vi "CTR_TCP_Init.vi"(6 "timeout ms":i32=-1, 8 "error in":errorcluster, 9 "port":u16, 10 "DAQ refDes":string, 11 "service name":string) -> (0 "error out":errorcluster, 1 "TCP Timeout":bool, 2 "Start DataStreams":bool=TRUE, 3 "connection ID":refnum<k5>)   [LabVIEW 2024]
panel:
  out "data out":string
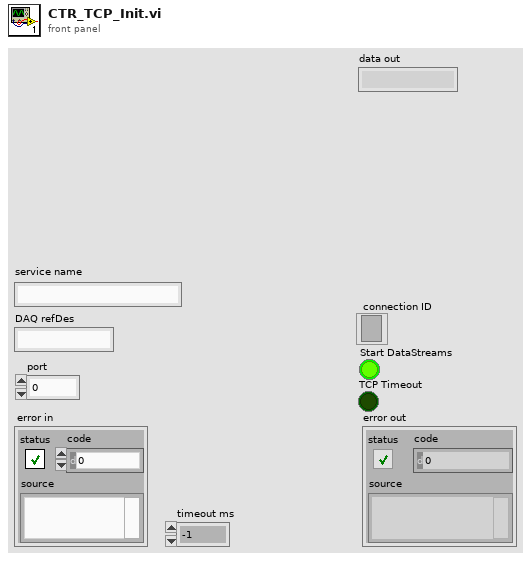
[diagram p1: front panel]
types:
  T1 = enum16{"Standard", "Buffered", "CRLF", "Immediate"}
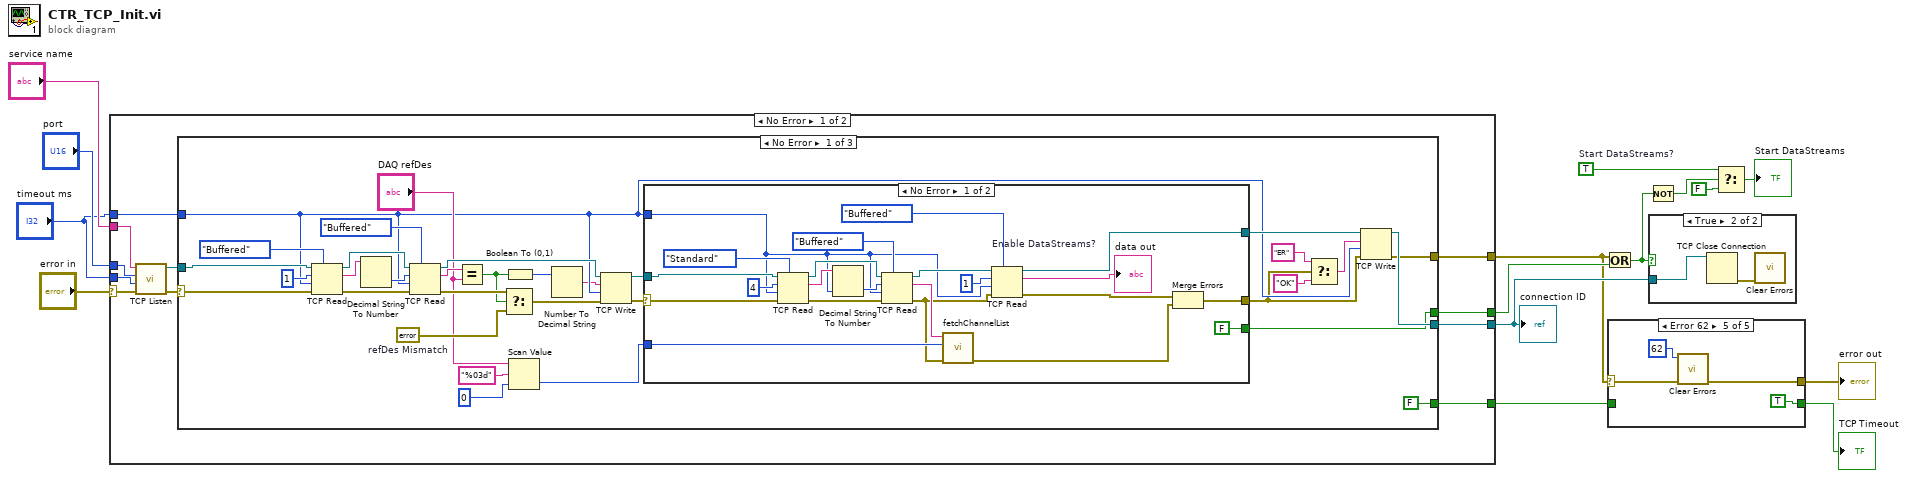
[diagram p0: block diagram]
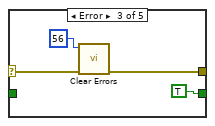
[diagram p4: hidden frame]
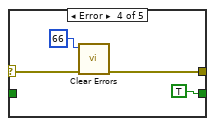
[diagram p5: hidden frame]
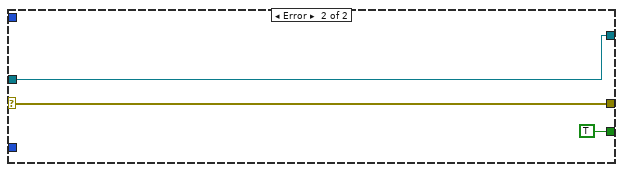
[diagram p7: hidden frame]
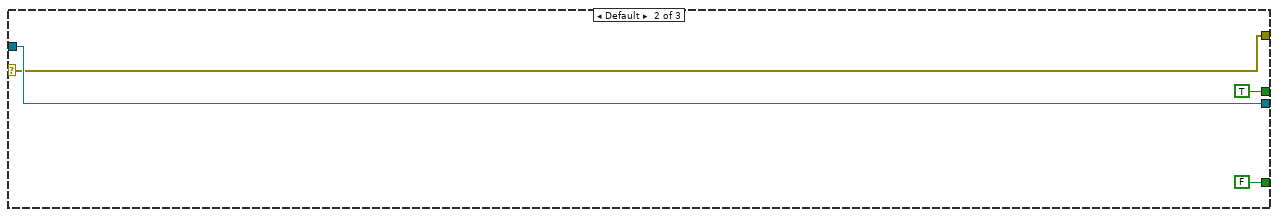
[diagram p8: hidden frame]
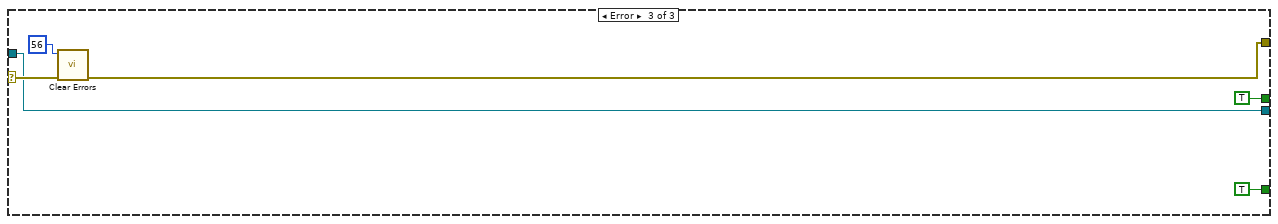
[diagram p9: hidden frame]
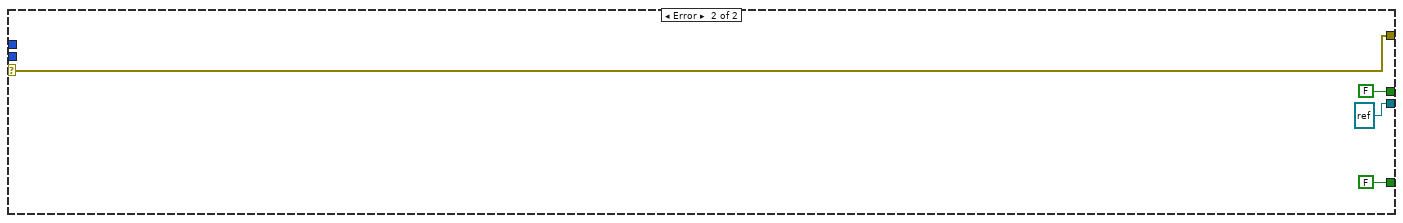
[diagram p10: hidden frame]
diagram:
  w13 = TRUE  # Start DataStreams?
  n1 = case shown="No Error" "error in" {
    selector: "error in" -> [w17 w98]
    tunnel: "service name" -> [w26 _]
    tunnel: "port" -> [w25 _]
    tunnel: [w23 refnum<k5> refnum ("connection ID")] -> w6
    tunnel: "timeout ms" -> [w22 _]
    tunnel: [w20 FALSE] -> w10
    tunnel: [w19 w98] -> w5
    tunnel: [w18 FALSE] -> w3
    tunnel: "timeout ms" -> [w16 _]
    frame No Error {
      n2 = call <vilib>:"TCP Listen.vi"("error in (no error)"=w17, "timeout ms (wait forever: -1)"=w22, "port"=w25, "service name"=w26) -> ("error out"=w21:errorcluster, "connection ID"=w24:refnum<k5>)  [unwired: 3 in, 3 out]
      n3 = case shown="No Error" w21 {
        selector: w21 -> [w30 w87 w94]
        tunnel: w24 -> [w59 w88 w91]
        tunnel: [w37 w88 w91] -> w23
        tunnel: [w36 w87 w92] -> w19
        tunnel: w16 -> [w35 _ _]
        tunnel: [w29 TRUE TRUE] -> w20
        tunnel: [FALSE FALSE TRUE] -> w18
        frame No Error {
          w50 = errorcluster {"status"=TRUE, "code"=0, "source"="refDes Mismatch"}  # refDes Mismatch
          n4 = TCP Read(connection ID=w59, bytes to read=1, error in (no error)=w30, 7:T1."Buffered" ("mode (standard)"), 9:w35) -> (connection ID out=w55:refnum<k5>, data out=w57:string, error out=w56:errorcluster)
          n5 = Decimal String To Number(string=w57) -> (number=w54:i32)  [unwired: 2 in, 1 out]
          n6 = TCP Read(connection ID=w55, bytes to read=w54, error in (no error)=w56, 7:T1."Buffered" ("mode (standard)"), 9:w35) -> (connection ID out=w48:refnum<k5>, data out=w52:string, error out=w51:errorcluster)
          n7 = Equal?(x=w52, y="DAQ refDes") -> (x = y?=w47:bool)
          n8 = Select(t=w51, s=w47, f=w50) -> (s? t:f=w49:errorcluster)
          n9 = Boolean To (0,1)(Boolean=w47) -> (0, 1=w46:i16)
          n10 = Scan Value(string="DAQ refDes", format string="%03d", default (0 dbl)=0) -> (value=w39:i32)  [unwired: 1 out]
          n11 = Number To Decimal String(number=w46) -> (decimal integer string=w27:string)  [unwired: 1 in]
          n12 = TCP Write(connection ID=w48, data in=w27, error in (no error)=w49, 9:w35) -> (connection ID out=w43:refnum<k5>, error out=w44:errorcluster)  [unwired: 1 out]
          n13 = case shown="No Error" w44 {
            selector: w44 -> [w61 w83]
            tunnel: w43 -> [w74 w84]
            tunnel: w35 -> [w60 _]
            tunnel: [w68 w83] -> w34
            tunnel: [w70 w84] -> w38
            tunnel: w39 -> [w72 _]
            tunnel: [FALSE TRUE] -> w29
            frame No Error {
              n14 = TCP Read(connection ID=w74, bytes to read=4, error in (no error)=w61, 7:T1."Standard" ("mode (standard)"), 9:w60) -> (connection ID out=w80:refnum<k5>, data out=w78:string, error out=w79:errorcluster)
              n15 = Decimal String To Number(string=w78, default (0L)=w60) -> (number=w81:i32)  [unwired: 1 in, 1 out]
              n16 = TCP Read(connection ID=w80, bytes to read=w81, error in (no error)=w79, 7:T1."Buffered" ("mode (standard)"), 9:w60) -> (connection ID out=w71:refnum<k5>, data out=w73:string, error out=w63:errorcluster)
              n17 = call "fetchChannelList.vi"("error in"=w63, "DAQ ID #"=w72, "Channels"=w73) -> ("error out"=w67:errorcluster)  [unwired: 6 in, 2 out]
              n18 = TCP Read "Enable DataStreams?"(connection ID=w71, bytes to read=1, error in (no error)=w63, 7:T1."Buffered" ("mode (standard)"), 9:w60) -> (connection ID out=w70:refnum<k5>, data out=→"data out":string, error out=w62:errorcluster)
              n19 = Merge Errors(w62, w67) -> (w68:errorcluster)
            }
            frame Error {
            }
          }
          n20 = Select(t="ER", s=w34, f="OK") -> (s? t:f=w31:string)
          n21 = TCP Write(connection ID=w38, data in=w31, error in (no error)=w34, 9:w35) -> (connection ID out=w37:refnum<k5>, error out=w36:errorcluster)  [unwired: 1 out]
        }
        frame Default {
        }
        frame Error {
          n22 = call <vilib>:"Clear Errors.vi"("error in (no error)"=w94, "specific error code to clear (0: all)"=56) -> ("error out"=w92:errorcluster)  [unwired: 4 in, 1 out]
        }
      }
    }
    frame Error {
    }
  }
  "connection ID" <- w6
  n23 = Or(x=w5, y=w10) -> (x .or. y?=w7:bool)
  n24 = case shown="Error 62" w5 {
    selector: w5 -> [w100 w102 w106 w110 w114]
    tunnel: [w100 w102 w104 w108 w112] -> w4
    tunnel: w3 -> [w99 w101 _ _ _]
    tunnel: [w99 w101 TRUE TRUE TRUE] -> w2
    frame No Error {
    }
    frame Default {
    }
    frame Error {
      n25 = call <vilib>:"Clear Errors.vi"("error in (no error)"=w106, "specific error code to clear (0: all)"=56) -> ("error out"=w104:errorcluster)  [unwired: 4 in, 1 out]
    }
    frame Error {
      n26 = call <vilib>:"Clear Errors.vi"("error in (no error)"=w110, "specific error code to clear (0: all)"=66) -> ("error out"=w108:errorcluster)  [unwired: 4 in, 1 out]
    }
    frame Error {
      n27 = call <vilib>:"Clear Errors.vi"("error in (no error)"=w114, "specific error code to clear (0: all)"=62) -> ("error out"=w112:errorcluster)  [unwired: 4 in, 1 out]
    }
  }
  "error out" <- w4
  "TCP Timeout" <- w2
  n28 = Not(x=w7) -> (.not. x?=w9:bool)
  n29 = case shown="True" w7 {
    tunnel: w6 -> [_ w116]
    frame False {
    }
    frame True {
      n30 = TCP Close Connection(connection ID=w116) -> (error out=w115:errorcluster)  [unwired: 2 in, 1 out]
      n31 = call <vilib>:"Clear Errors.vi"("error in (no error)"=w115) -> ()  [unwired: 5 in, 2 out]
    }
  }
  n32 = Select(t=w13, s=w9, f=FALSE) -> (s? t:f=→"Start DataStreams":bool)
